vi "Save.vi"(7 "source paths":path[](array[path]), 8 "error in (no error)":errorcluster, 10 "processed sources":refnum<class "AB_Source.lvclass">[](array[class]), 11 "AB_PackedLibrary in":refnum<class "AB_PackedLibrary.lvclass">) -> (0 "error out":errorcluster, 1 "TypeInfo":string, 2 "source destination paths":path[](array[path]), 3 "AB_PackedLibrary out":refnum<class "AB_PackedLibrary.lvclass">, 4 "eng_LEIFBuildData":u32, 5 "checksums":string[](array[string]))   [LabVIEW 2020, in "AB_PackedLibrary.lvclass"]
uses:
  <vilib>/AppBuilder/AB_Classes/PackedLib/AB_PackedLibrary.lvclass
  e:/builds/penguin/labview/branches/2020/dev/dist/vi.lib/AppBuilder/AB_Classes/TargetFile/AB_Targetfile.lvclass
  e:/builds/penguin/labview/branches/2020/dev/dist/vi.lib/AppBuilder/AB_Classes/Build/AB_Build.lvclass
  <vilib>/AppBuilder/AB_Classes/Source/AB_Source.lvclass
  <vilib>/AppBuilder/AB_Classes/TargetFile/AB_Targetfile.lvclass
  <vilib>/AppBuilder/AB_Classes/Build/AB_Build.lvclass
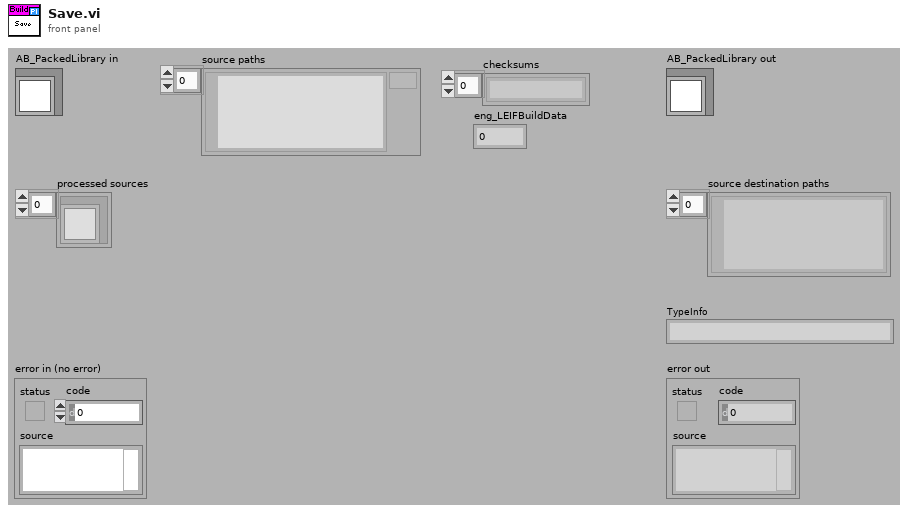
[diagram p1: front panel]
types:
  T1 = typedef "AB_Log_Save_Action.ctl" = enum32{"consolidated save with types", "consolidated save", "save"}
  T2 = typedef "AB_Targetfile.ctl" = cluster{"targetfileName":string, "targetfileGUID":string, "enableDebugging":bool, "versionInfo":cluster{"productName":string, "legalCopyright":string, "companyName":string, "internalName":string, "fileDescription":string}, "eng_consolidatedTypeInfo":string, "fastFileFormat":bool, "eng_LEIFBuildData":u32, "versionIndependent":bool}
  T3 = typedef "AB_Build.ctl" = cluster{"buildSpecName":string, "buildSpecDescription":string, "destinations":refnum<class "AB_Destination.lvclass">[], "exclusionOption":T4, "defaultLanguage":string, "supportedLanguages":string[], "excludedDirectories":path[], "buildContext":refnum<vi>, "buildObject":T5, "preview":bool, "programatic":bool, "progressBarEvents":T6, "userLog_Path":path, "preActionID":string, "preAction_Path":path, "postActionID":string, "postAction_Path":path, "eng_checkForBrokenVIs?":bool, "eng_verboseLinkerErrors?":bool, "localDest_Path":path, "targetDest_Path":path, "removeVIObject":u16, "cache":refnum<class "PreviewCache.lvclass">, "use cache":bool, "previewCache_ID":string, "buildCache_ID":string, "eng_TempLocalDest_Path":path, "eng_collectDependencies?":bool, "versionInfo":cluster{"buildVersion":cluster{"major":u16, "minor":u16, "patch":u16, "build":u16}, "autoIncrement":bool}, "eng_enableVIChecksums":bool}
  T4 = typedef "AB_Exclusion_Option.ctl" = cluster{"typedefs":bool, "polymorphicVIs":bool, "unusedLibraryItems":bool, "modifyLibraryFile":bool, "edit-timeDependencies":bool, "inlineVIs":bool, "dependent PPLs":bool, "dependent DLLs":bool}
  T5 = typedef "ItemRef.ctl" = u64
  T6 = typedef "provcom_ProgressBar_Events.ctl" = cluster{"newJob":refnum<user-event>, "newItem":refnum<user-event>, "errorMsg":T7, "cancel":refnum<user-event>}
  T7 = typedef "mxLvBuildError.ctl" = refnum<user-event>
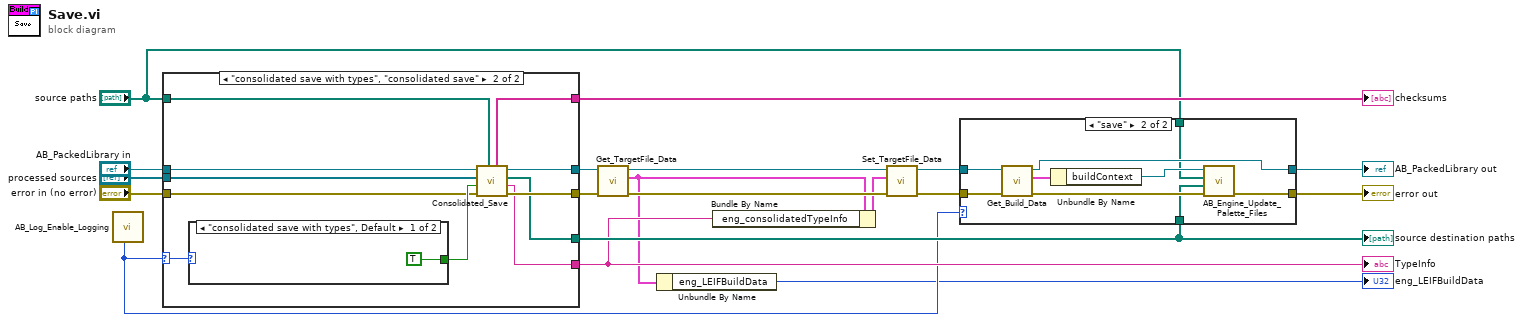
[diagram p0: block diagram]
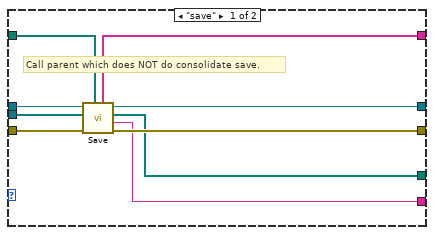
[diagram p3: hidden frame]
diagram:
  n1 = call <vilib>:"AB_Log_Enable_Logging.vi"() -> ("save mode"=w3:T1)  [unwired: 4 in, 7 out]
  n2 = case shown="\"consolidated save with types\", \"consolidated save\"" w3 {
    selector: w3 -> [_ w39]
    tunnel: "processed sources" -> [w24 w33]
    tunnel: "error in (no error)" -> [w23 w31]
    tunnel: [w27 w37] -> w5
    tunnel: [w28 w38] -> w7
    tunnel: [w21 w29] -> w4
    tunnel: "source paths" -> [w22 w32]
    tunnel: [w26 w30] -> w13
    tunnel: "AB_PackedLibrary in" -> [w25 w34]
    tunnel: [w20 w36] -> w14
    frame "save" {
      # "Call parent which does NOT do consolidate save."
      n3 = call-parent "Save.vi"("source paths"=w22, "error in"=w23, "processed sources"=w24, "AB_Build in"=w25) -> ("error out"=w27:errorcluster, "TypeInfo"=w21:string, "source destination paths"=w26:path[], "AB_Build out"=w28:refnum<class "AB_PackedLibrary.lvclass">, "checksums"=w20:string[])  [unwired: 2 in, 1 out]
    }
    frame "consolidated save with types", "consolidated save" {
      n4 = case shown="\"consolidated save with types\", Default" w39 {
        tunnel: [TRUE _] -> w35
        frame "consolidated save with types", Default {
        }
        frame "consolidated save" {
        }
      }
      n5 = call <vilib>:"Consolidated_Save.vi"("source paths"=w32, "error in"=w31, "Use Consolidated Types"=w35, "processed sources"=w33, "AB_Targetfile in"=w34) -> ("error out"=w37:errorcluster, "TypeInfo"=w29:string, "source destination paths"=w30:path[], "AB_Targetfile out"=w38:refnum<class "AB_PackedLibrary.lvclass">, "checksums"=w36:string[])  [unwired: 2 in]
    }
  }
  "source destination paths" <- w13
  "TypeInfo" <- w4
  "checksums" <- w14
  n6 = call <vilib>:"Get_TargetFile_Data.vi"("error in (no error)"=w5, "AB_Targetfile in"=w7) -> ("error out"=w10:errorcluster, "data"=w2:T2, "AB_Targetfile out"=w11:refnum<class "AB_PackedLibrary.lvclass">)  [unwired: 7 in]
  n7 = Unbundle By Name(w2) -> ("eng_LEIFBuildData"=→"eng_LEIFBuildData":u32)
  n8 = Bundle By Name(cluster=w2, "eng_consolidatedTypeInfo"=w4) -> (w9:T2)
  n9 = call <vilib>:"Set_TargetFile_Data.vi"("error in (no error)"=w10, "data"=w9, "AB_Targetfile in"=w11) -> ("error out"=w6:errorcluster, "AB_Targetfile out"=w8:refnum<class "AB_PackedLibrary.lvclass">)  [unwired: 7 in]
  n10 = case shown="\"save\"" w3 {
    tunnel: [w41 w51] -> w17
    tunnel: [w42 w49] -> w16
    tunnel: w13 -> [_ w46]
    tunnel: "source paths" -> [_ w45]
    tunnel: w8 -> [w42 w44]
    tunnel: w6 -> [w41 w43]
    frame "consolidated save with types", "consolidated save" {
    }
    frame "save" {
      n11 = call <vilib>:"Get_Build_Data.vi"("error in (no error)"=w43, "Class in"=w44) -> ("error out"=w50:errorcluster, "data"=w48:T3, "Class out"=w49:refnum<class "AB_PackedLibrary.lvclass">)  [unwired: 7 in]
      n12 = Unbundle By Name(w48) -> ("buildContext"=w47:refnum<vi>)
      n13 = call <vilib>:"AB_Engine_Update_Palette_Files.vi"("error in"=w50, "new paths"=w46, "old paths"=w45, "application reference"=w47) -> ("error out"=w51:errorcluster)  [unwired: 7 in]
    }
  }
  "error out" <- w17
  "AB_PackedLibrary out" <- w16
